vi "Udpate Task Display Name.vi"(8 "error in (no error)":errorcluster, 9 "Display Name":string, 10 "Task":i32, 11 "Task Setting Editor in":refnum<class "Task Setting Editor.lvclass">) -> (0 "error out":errorcluster, 3 "Task Setting Editor out":refnum<class "Task Setting Editor.lvclass">)   [LabVIEW 2017, in "Task Setting Editor.lvlib" / "Task Setting Editor.lvclass"]
uses:
  Task Setting Editor.lvclass
  Task Setting Editor.lvclass/Task Setting Editor.ctl
  BuildWorker/Classes/Task/Task.lvclass/Task.ctl
  BuildWorker/Classes/Task/Write Display Name.vi
  BuildWorker/Classes/Task/Task.lvclass
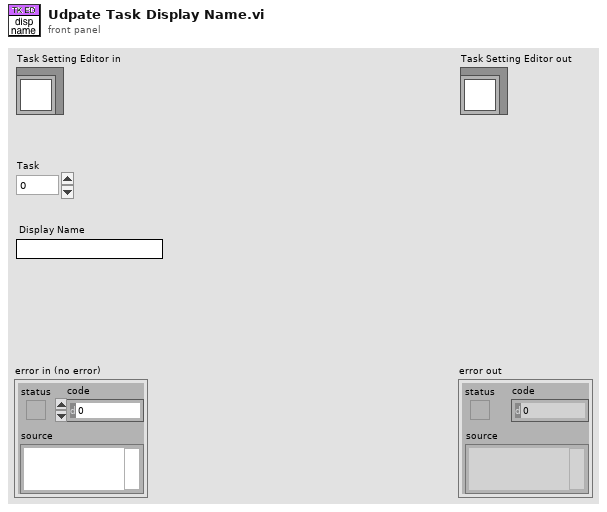
[diagram p1: front panel]
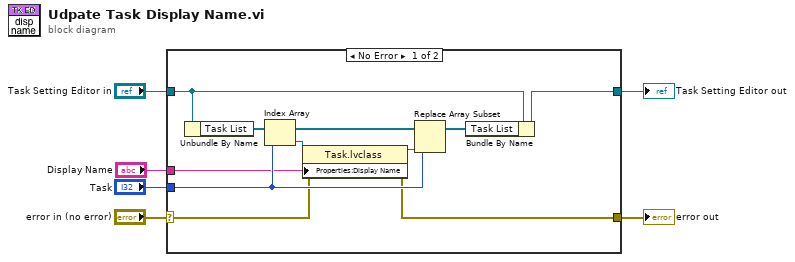
[diagram p0: block diagram]
diagram:
  n1 = case shown="No Error" "error in (no error)" {
    selector: "error in (no error)" -> [w10 w18]
    tunnel: [w9 w18] -> w5
    tunnel: [w8 w17] -> w3
    tunnel: "Task Setting Editor in" -> [w16 w17]
    tunnel: "Display Name" -> [w11 _]
    tunnel: "Task" -> [w14 _]
    frame No Error {
      n2 = Unbundle By Name(w16) -> ("Task List"=w15:refnum<class "Task.lvclass">[])
      n3 = Index Array(array=w15, index=w14) -> (element=w13:refnum<class "Task.lvclass">)
      n4 = property class="Task.lvclass"(reference=w13, error in=w10, "Properties:Display Name"=w11) -> (reference out=w12:refnum<class "Task.lvclass">, error out=w9:errorcluster)
      n5 = Replace Array Subset(array=w15, new element=w12, index=w14) -> (w7:refnum<class "Task.lvclass">[])
      n6 = Bundle By Name(cluster=w16, "Task List"=w7) -> (w8:refnum<class "Task Setting Editor.lvclass">)
    }
    frame Error {
    }
  }
  "error out" <- w5
  "Task Setting Editor out" <- w3
